vi "Auto State Machine.vi"(8 "Scale":string, 9 "Switch":string, 10 "index of element":i32, 11 "Starting Position":T1) -> ()   [LabVIEW 2017]
uses:
  Support Code/Starting Position.ctl
  <vilib>/Rock Robotics/WPI/Framework/Command Status Info.ctl
  <vilib>/Rock Robotics/WPI/Framework/Completion Status.ctl
  <vilib>/Rock Robotics/WPI/Framework/Completion Notifier.ctl
  Block Clusters/Far--L.ctl
  Block Clusters/L--end Sw.ctl
  Block Clusters/end Sw--sq C1.ctl
  Block Clusters/C1--d Hi.ctl
  Block Clusters/C1--C3.ctl
  Block Clusters/C3--C4.ctl
  Block Clusters/d Hi--C1.ctl
  Block Clusters/C3--End Sw.ctl
  Block Clusters/front Sw--L.ctl
  Block Clusters/C3--cube Sw.ctl
  Block Clusters/M--front LSw.ctl
  Block Clusters/M--front RSw.ctl
  Block Clusters/end cube--C1.ctl
  Block Clusters/C1--end cube.ctl
  Block Clusters/L--C1.ctl
  Block Clusters/SQ Hi--C1.ctl
  Block Clusters/C1--sq Hi.ctl
  Block Clusters/front Sw--P cube1.ctl
  Block Clusters/P cube1--front Sw.ctl
  Framework/Robot Global Data.vi
  <vilib>/Rock Robotics/Network Tables/NT Write String Array.vi
  <vilib>/Rock Robotics/Network Tables/NT Write String.vi
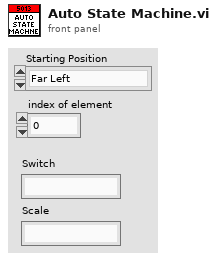
[diagram p1: front panel]
types:
  T1 = typedef "Starting Position.ctl" = enum16{"Far Left", "Middle", "Far Right"}
  T2 = typedef "Command Status Info.ctl" = cluster{"Name":string, "Status":T3, "notifier out":T4}
  T3 = typedef "Completion Status.ctl" = enum16{"Successful", "Aborted", "Incomplete"}
  T4 = typedef "Completion Notifier.ctl" = refnum<notifier>
  T5 = typedef "Routines and Block Data.ctl" = cluster{"Routines":T6[][], "Block Data Array":variant[]}
  T6 = typedef "Blocks.ctl" = enum16{"", "Wait 1s", "Far--L", "L--end Sw", "end Sw--sq C1", "end cube--C1", "C1--d Hi", "C1--C3", "C3--C4", "d Hi--C1", "C3--end Sw", "C3--cube Sw", "M--front LSw", "M--front RSw", "front Sw--L", "L--C1", "C1--end cube", "sq Hi--C1", "C1--sq Hi", "front Sw--P cube1", "P cube1--front Sw"}
  T7 = typedef "Far--L.ctl" = cluster{"1a":dbl, "1d":dbl, "1s":dbl}
  T8 = typedef "L--end Sw.ctl" = cluster{"1d":dbl, "1s":dbl, "2t":dbl, "3a":dbl, "4d":dbl, "4s":dbl}
  T9 = typedef "end Sw--sq C1.ctl" = cluster{"1a":dbl, "1d":dbl, "1s":dbl, "2d":dbl, "2s":dbl}
  T10 = typedef "C1--d Hi.ctl" = cluster{"1t":dbl, "2d":dbl, "2s":dbl, "3a":dbl, "4d":dbl, "4s":dbl}
  T11 = typedef "C1--C3.ctl" = cluster{"1a":dbl, "2d":dbl, "2s":dbl}
  T12 = typedef "C3--C4.ctl" = cluster{"1a":dbl, "1d":dbl, "1s":dbl}
  T13 = typedef "d Hi--C1.ctl" = cluster{"1a":dbl, "1d":dbl, "1s":dbl, "3t":dbl, "4d":dbl, "4s":dbl}
  T14 = typedef "C3--End Sw.ctl" = cluster{"1a":dbl, "1d":dbl, "1s":dbl, "2a":dbl, "3t":dbl, "4d":dbl, "4s":dbl, "5a":dbl, "6d":dbl, "6s":dbl}
  T15 = typedef "front Sw--L.ctl" = cluster{"1d":dbl, "1s":dbl, "2a":dbl, "3t":dbl, "4d":dbl, "4s":dbl, "5a":dbl}
  T16 = typedef "C3--cube Sw.ctl" = cluster{"1a":dbl, "1d":dbl, "1s":dbl, "2a":dbl, "4d":dbl, "4s":dbl, "5t":dbl}
  T17 = typedef "M--front LSw.ctl" = cluster{"1d":dbl, "1s":dbl, "2a":dbl, "3t":dbl, "4d":dbl, "4s":dbl, "5a":dbl, "6d":dbl, "6s":dbl}
  T18 = typedef "M--front RSw.ctl" = cluster{"1a":dbl, "1d":dbl, "1s":dbl}
  T19 = typedef "end cube--C1.ctl" = cluster{"1a":dbl, "1d":dbl, "1s":dbl, "2a":dbl}
  T20 = typedef "C1--end cube.ctl" = cluster{"1a":dbl, "2d":dbl, "2s":dbl, "3g":dbl, "4t":dbl}
  T21 = typedef "L--C1.ctl" = cluster{"1a":dbl, "1d":dbl, "1s":dbl}
  T22 = typedef "SQ Hi--C1.ctl" = cluster{"1a":dbl, "1d":dbl, "1s":dbl, "2d":dbl, "2s":dbl}
  T23 = typedef "C1--sq Hi.ctl" = cluster{"1d":dbl, "1s":dbl, "2a":dbl, "2d":dbl, "2s":dbl}
  T24 = typedef "front Sw--P cube1.ctl" = cluster{"1a":dbl, "1d":dbl, "1s":dbl, "2a":dbl, "2d":dbl, "2s":dbl, "3d":dbl, "3s":dbl, "1t":dbl}
  T25 = typedef "P cube1--front Sw.ctl" = cluster{"1a":dbl, "1d":dbl, "1s":dbl, "2a":dbl, "1t":dbl, "2d":dbl, "2s":dbl, "3d":dbl, "3s":dbl}
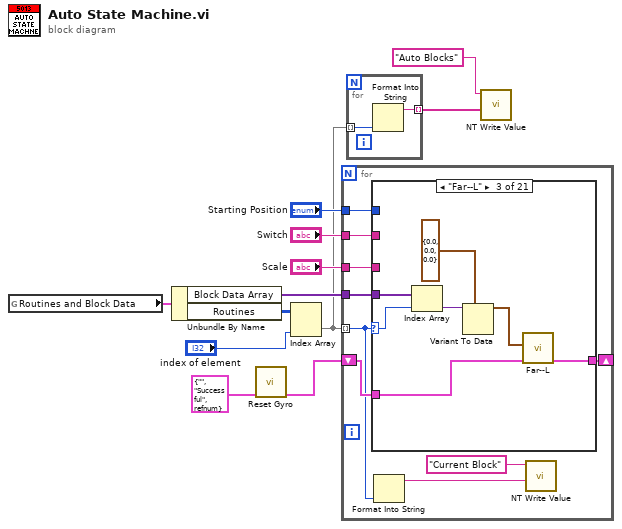
[diagram p0: block diagram]
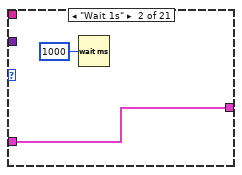
[diagram p3: hidden frame]
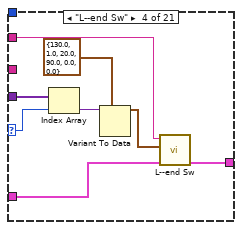
[diagram p4: hidden frame]
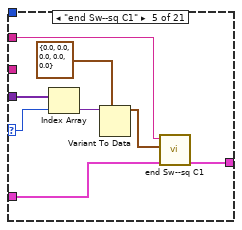
[diagram p5: hidden frame]
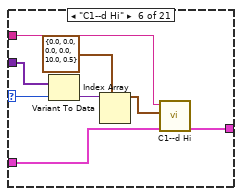
[diagram p6: hidden frame]
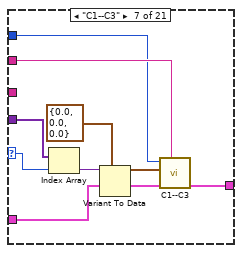
[diagram p7: hidden frame]
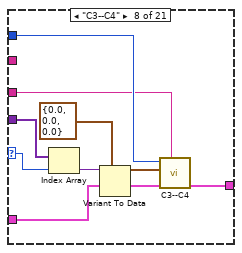
[diagram p8: hidden frame]
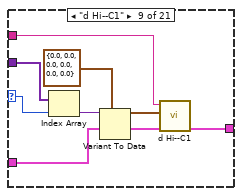
[diagram p9: hidden frame]
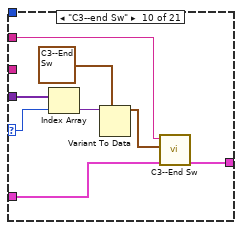
[diagram p10: hidden frame]
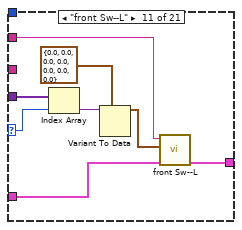
[diagram p11: hidden frame]
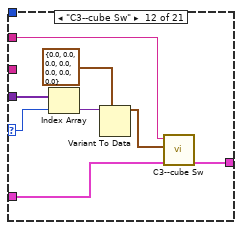
[diagram p12: hidden frame]
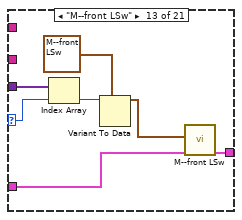
[diagram p13: hidden frame]
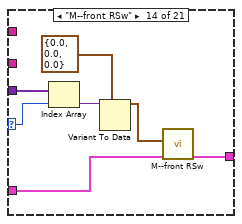
[diagram p14: hidden frame]
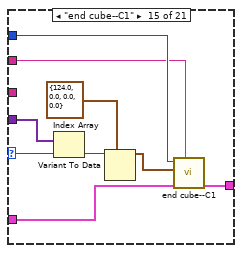
[diagram p15: hidden frame]
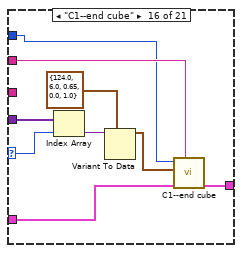
[diagram p16: hidden frame]
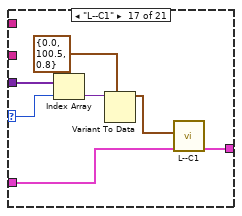
[diagram p17: hidden frame]
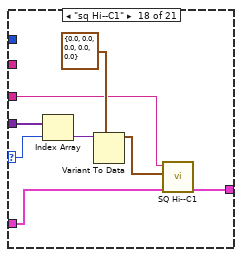
[diagram p18: hidden frame]
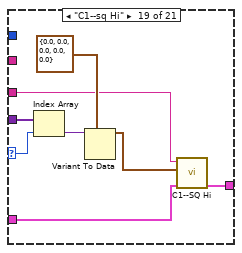
[diagram p19: hidden frame]
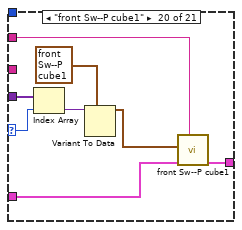
[diagram p20: hidden frame]
diagram:
  n1 = global read "Robot Global Data.vi" "Routines and Block Data"() -> (w11:T5)
  n2 = Unbundle By Name(w11) -> ("Block Data Array"=w10:variant[], "Routines"=w12:T6[][])
  n3 = call "Reset Gyro.vi"("Command Info In"=T2 {"Name"="", "Status"=enum."Successful", "notifier out"=refnum}) -> ("Command Info Out"=w5:T2)  [unwired: 10 in]
  n4 = Index Array(array=w12, index (col)="index of element") -> (element=w3:T6[])  [unwired: 1 in]
  n5 = for {
    tunnel: w3 -> [w13] mode=indexing
    tunnel: w10 -> [w21]
    shift-right: [w19] -> _
    shift-left: w5 -> [w20]
    tunnel: "Switch" -> [w18]
    tunnel: "Scale" -> [w17]
    tunnel: "Starting Position" -> [w16]
    n6 = case shown="\"Far--L\"" w13 {
      selector: w13 -> [_ _ w30 w38 w46 w54 w63 w72 w80 w88 w96 w104 w111 w118 w127 w136 w143 w150 w156 w166 w175]
      tunnel: w21 -> [_ _ w31 w39 w47 w55 w64 w73 w81 w89 w97 w105 w112 w119 w128 w137 w144 w151 w157 w167 w174]
      tunnel: w20 -> [w22 w23 w26 w36 w44 w52 w61 w70 w78 w86 w94 w102 w106 w115 w124 w133 w141 w148 w159 w164 w171]
      tunnel: [w22 w23 w25 w35 w43 w51 w60 w69 w77 w85 w93 w101 w109 w114 w123 w132 w140 w147 w160 w163 w172] -> w19
      tunnel: w18 -> [_ _ _ w32 w40 _ w57 _ _ w84 w92 w98 _ _ w120 w130 _ _ _ w162 w169]
      tunnel: w17 -> [_ _ _ _ _ w48 _ w65 w74 _ _ _ _ _ _ _ _ w145 w153 _ _]
      tunnel: w16 -> [_ _ _ _ _ _ w56 w66 _ _ _ _ _ _ w121 w129 _ _ _ _ _]
      frame "" {
      }
      frame "Wait 1s" {
        n7 = Wait (ms)(milliseconds to wait=u32 1000) -> ()  [unwired: 1 out]
      }
      frame "Far--L" {
        n8 = Index Array(array=w31, index=w30) -> (element=w29:variant)
        n9 = Variant To Data(type=T7 {"1a"=0.0, "1d"=0.0, "1s"=0.0} ("Far to Line1"), Variant=w29) -> (data=w27:T7)  [unwired: 1 in, 1 out]
        n10 = call "Far--L.vi"("Command Info In"=w26, "Far--L"=w27) -> ("Command Info Out"=w25:T2)  [unwired: 7 in]
      }
      frame "L--end Sw" {
        n11 = Index Array(array=w39, index=w38) -> (element=w37:variant)
        n12 = Variant To Data(type=T8 {"1d"=130.0, "1s"=1.0, "2t"=20.0, "3a"=90.0, "4d"=0.0, "4s"=0.0} ("Line1 to ESwitch1"), Variant=w37) -> (data=w33:T8)  [unwired: 1 in, 1 out]
        n13 = call "L--end Sw.vi"("Command Info In"=w36, "L--end Sw"=w33, "Switch"=w32) -> ("Command Info Out"=w35:T2)  [unwired: 6 in]
      }
      frame "end Sw--sq C1" {
        n14 = Index Array(array=w47, index=w46) -> (element=w45:variant)
        n15 = Variant To Data(type=T9 {"1a"=0.0, "1d"=0.0, "1s"=0.0, "2d"=0.0, "2s"=0.0} ("End Switch To Corridor"), Variant=w45) -> (data=w41:T9)  [unwired: 1 in, 1 out]
        n16 = call "end Sw--sq C1.vi"("Command Info In"=w44, "end Sw--sq C1"=w41, "Switch"=w40) -> ("Command Info Out"=w43:T2)  [unwired: 8 in]
      }
      frame "C1--d Hi" {
        n17 = Index Array(array=w55, index=w54) -> (element=w53:variant)
        n18 = Variant To Data(type=T10 {"1t"=0.0, "2d"=0.0, "2s"=0.0, "3a"=0.0, "4d"=10.0, "4s"=0.5} ("Corridor to Diag Scale"), Variant=w53) -> (data=w49:T10)  [unwired: 1 in, 1 out]
        n19 = call "C1--d Hi.vi"("Command Info In"=w52, "Corridor to Diag Scale"=w49, "Scale"=w48) -> ("Command Info Out"=w51:T2)  [unwired: 8 in]
      }
      frame "C1--C3" {
        n20 = Index Array(array=w64, index=w63) -> (element=w62:variant)
        n21 = Variant To Data(type=T11 {"1a"=0.0, "2d"=0.0, "2s"=0.0} ("C1 to C3"), Variant=w62) -> (data=w58:T11)  [unwired: 1 in, 1 out]
        n22 = call "C1--C3.vi"("Starting Position"=w56, "C1--C3"=w58, "Command Info In"=w61, "Switch"=w57) -> ("Command Info Out"=w60:T2)  [unwired: 6 in]
      }
      frame "C3--C4" {
        n23 = Index Array(array=w73, index=w72) -> (element=w71:variant)
        n24 = Variant To Data(type=T12 {"1a"=0.0, "1d"=0.0, "1s"=0.0} ("C3 to C4"), Variant=w71) -> (data=w67:T12)  [unwired: 1 in, 1 out]
        n25 = call "C3--C4.vi"("Scale"=w65, "Command Info In"=w70, "C3 to C4"=w67, "Starting Position"=w66) -> ("Command Info Out"=w69:T2)  [unwired: 7 in]
      }
      frame "d Hi--C1" {
        n26 = Index Array(array=w81, index=w80) -> (element=w79:variant)
        n27 = Variant To Data(type=T13 {"1a"=0.0, "1d"=0.0, "1s"=0.0, "3t"=0.0, "4d"=0.0, "4s"=0.0} ("Block Inputs"), Variant=w79) -> (data=w75:T13)  [unwired: 1 in, 1 out]
        n28 = call "d Hi--C1.vi"("Command Info In"=w78, "d Hi--C1"=w75, "Scale"=w74) -> ("Command Info Out"=w77:T2)  [unwired: 8 in]
      }
      frame "C3--end Sw" {
        n29 = Index Array(array=w89, index=w88) -> (element=w87:variant)
        n30 = Variant To Data(type=T14 {"1a"=0.0, "1d"=0.0, "1s"=0.0, "2a"=0.0, "3t"=0.0, "4d"=0.0, "4s"=0.0, "5a"=0.0, "6d"=0.0, "6s"=0.0} ("Block Inputs"), Variant=w87) -> (data=w82:T14)  [unwired: 1 in, 1 out]
        n31 = call "C3--End Sw.vi"("Command Info In"=w86, "C3--End Sw"=w82, "Switch"=w84) -> ("Command Info Out"=w85:T2)  [unwired: 8 in]
      }
      frame "front Sw--L" {
        n32 = Index Array(array=w97, index=w96) -> (element=w95:variant)
        n33 = Variant To Data(type=T15 {"1d"=0.0, "1s"=0.0, "2a"=0.0, "3t"=0.0, "4d"=0.0, "4s"=0.0, "5a"=0.0} ("front Sw--L"), Variant=w95) -> (data=w91:T15)  [unwired: 1 in, 1 out]
        n34 = call "front Sw--L.vi"("Command Info In"=w94, "F-SW--Line"=w91, "Switch"=w92) -> ("Command Info Out"=w93:T2)  [unwired: 8 in]
      }
      frame "C3--cube Sw" {
        n35 = Index Array(array=w105, index=w104) -> (element=w103:variant)
        n36 = Variant To Data(type=T16 {"1a"=0.0, "1d"=0.0, "1s"=0.0, "2a"=0.0, "4d"=0.0, "4s"=0.0, "5t"=0.0} ("C3 to Cube and Switch"), Variant=w103) -> (data=w99:T16)  [unwired: 1 in, 1 out]
        n37 = call "C3--cube Sw.vi"("Command Info In"=w102, "C3--cube Sw"=w99, "Switch"=w98) -> ("Command Info Out"=w101:T2)  [unwired: 8 in]
      }
      frame "M--front LSw" {
        n38 = Index Array(array=w112, index=w111) -> (element=w110:variant)
        n39 = Variant To Data(type=T17 {"1d"=0.0, "1s"=0.0, "2a"=0.0, "3t"=0.0, "4d"=0.0, "4s"=0.0, "5a"=0.0, "6d"=0.0, "6s"=0.0} ("M--front LSw"), Variant=w110) -> (data=w107:T17)  [unwired: 1 in, 1 out]
        n40 = call "M--front LSw.vi"("Command Info In"=w106, "M--front LSw"=w107) -> ("Command Info Out"=w109:T2)  [unwired: 9 in]
      }
      frame "M--front RSw" {
        n41 = Index Array(array=w119, index=w118) -> (element=w117:variant)
        n42 = Variant To Data(type=T18 {"1a"=0.0, "1d"=0.0, "1s"=0.0} ("M--front RSw"), Variant=w117) -> (data=w113:T18)  [unwired: 1 in, 1 out]
        n43 = call "M--front RSw.vi"("Command Info In"=w115, "M--front RSw"=w113) -> ("Command Info Out"=w114:T2)  [unwired: 9 in]
      }
      frame "end cube--C1" {
        n44 = Index Array(array=w128, index=w127) -> (element=w126:variant)
        n45 = Variant To Data(type=T19 {"1a"=124.0, "1d"=0.0, "1s"=0.0, "2a"=0.0} ("end cube--C1"), Variant=w126) -> (data=w122:T19)  [unwired: 1 in, 1 out]
        n46 = call "end cube--C1.vi"("Switch"=w120, "Command Info In"=w124, "end cube--C1"=w122, "Starting Position"=w121) -> ("Command Info Out"=w123:T2)  [unwired: 7 in]
      }
      frame "C1--end cube" {
        n47 = Index Array(array=w137, index=w136) -> (element=w135:variant)
        n48 = Variant To Data(type=T20 {"1a"=124.0, "2d"=6.0, "2s"=0.65, "3g"=0.0, "4t"=1.0} ("Block Inputs"), Variant=w135) -> (data=w131:T20)  [unwired: 1 in, 1 out]
        n49 = call "C1--end cube.vi"("Switch"=w130, "Command Info In"=w133, "C1--end cube"=w131, "Starting Position"=w129) -> ("Command Info Out"=w132:T2)  [unwired: 7 in]
      }
      frame "L--C1" {
        n50 = Index Array(array=w144, index=w143) -> (element=w142:variant)
        n51 = Variant To Data(type=T21 {"1a"=0.0, "1d"=100.5, "1s"=0.8} ("L--C1"), Variant=w142) -> (data=w139:T21)  [unwired: 1 in, 1 out]
        n52 = call "L--C1.vi"("Command Info In"=w141, "L--C1"=w139) -> ("Command Info Out"=w140:T2)  [unwired: 7 in]
      }
      frame "sq Hi--C1" {
        n53 = Index Array(array=w151, index=w150) -> (element=w152:variant)
        n54 = Variant To Data(type=T22 {"1a"=0.0, "1d"=0.0, "1s"=0.0, "2d"=0.0, "2s"=0.0} ("sq Hi--C1"), Variant=w152) -> (data=w146:T22)  [unwired: 1 in, 1 out]
        n55 = call "SQ Hi--C1.vi"("Command Info In"=w148, "Sq. Hi--C1"=w146, "Scale"=w145) -> ("Command Info Out"=w147:T2)  [unwired: 8 in]
      }
      frame "C1--sq Hi" {
        n56 = Index Array(array=w157, index=w156) -> (element=w158:variant)
        n57 = Variant To Data(type=T23 {"1d"=0.0, "1s"=0.0, "2a"=0.0, "2d"=0.0, "2s"=0.0} ("output cluster"), Variant=w158) -> (data=w155:T23)  [unwired: 1 in, 1 out]
        n58 = call "C1--SQ Hi.vi"("Command Info In"=w159, "C1--S Hi"=w155, "Scale"=w153) -> ("Command Info Out"=w160:T2)  [unwired: 8 in]
      }
      frame "front Sw--P cube1" {
        n59 = Index Array(array=w167, index=w166) -> (element=w168:variant)
        n60 = Variant To Data(type=T24 {"1a"=0.0, "1d"=0.0, "1s"=0.0, "2a"=0.0, "2d"=0.0, "2s"=0.0, "3d"=0.0, "3s"=0.0, "1t"=0.0} ("output cluster"), Variant=w168) -> (data=w161:T24)  [unwired: 1 in, 1 out]
        n61 = call "front Sw--P cube1.vi"("F-Sw--F-Cube"=w161, "Command Info In"=w164, "Switch"=w162) -> ("Command Info Out"=w163:T2)  [unwired: 7 in]
      }
      frame "P cube1--front Sw" {
        n62 = Index Array(array=w174, index=w175) -> (element=w176:variant)
        n63 = Variant To Data(type=T25 {"1a"=0.0, "1d"=40.0, "1s"=-0.85, "2a"=-90.0, "1t"=3.0, "2d"=57.0, "2s"=1.0, "3d"=81.0, "3s"=0.65} ("Block Inputs"), Variant=w176) -> (data=w170:T25)  [unwired: 1 in, 1 out]
        n64 = call "P cube1--front Sw.vi"("P Cube1--front sw"=w170, "Command Info In"=w171, "Switch"=w169) -> ("Command Info Out"=w172:T2)  [unwired: 7 in]
      }
    }
    n65 = Format Into String(w13) -> (resulting string=w15:string)  [unwired: 3 in, 1 out]
    n66 = call-poly <vilib>:"NT Write Value.vi"("String"=w15, "Name"="Current Block") -> ()  [unwired: 9 in, 1 out]
  }
  n67 = for {
    tunnel: w3 -> [w178] mode=indexing
    tunnel: [w177] -> w2 mode=indexing
    n68 = Format Into String(w178) -> (resulting string=w177:string)  [unwired: 3 in, 1 out]
  }
  n69 = call-poly <vilib>:"NT Write Value.vi"("String Array"=w2, "Name"="Auto Blocks") -> ()  [unwired: 9 in, 1 out]
